vi "Additional config for txt file.vi"() -> (0 "Configuration for text file":T1)   [LabVIEW 2017]
panel:
  in  "Sweep duration (sec)":dbl=20000.0
  in  "정지":bool
  in  "Baseline Offset (pA)":dbl
  in  "Unit (A or pA)":u16(ring) items=["A", "pA"]
  in  "Sampling rate (Hz)":dbl=20000.0
  # "Please enter additional information about the data file"
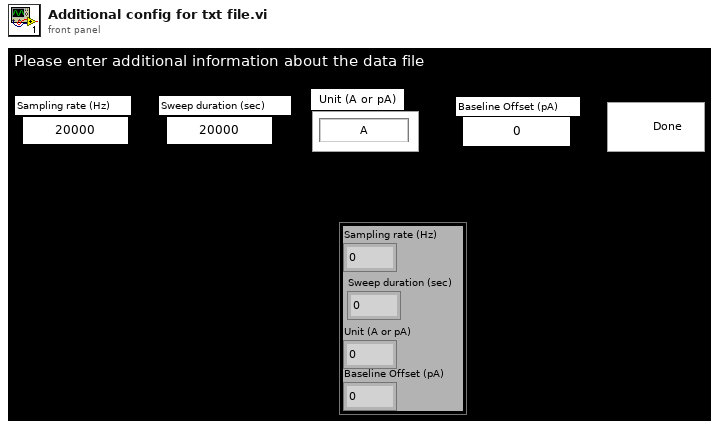
[diagram p1: front panel]
types:
  T1 = cluster{"Sampling rate (Hz)":dbl, "Sweep duration (sec)":dbl, "Unit (A or pA)":u16, "Baseline Offset (pA)":dbl}
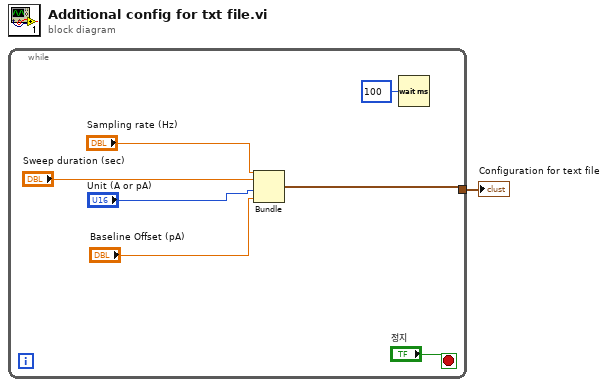
[diagram p0: block diagram]
diagram:
  n1 = while {
    tunnel: [w6] -> w1
    stop <- "정지" stop-if-true
    n2 = Bundle("Sampling rate (Hz)"="Sampling rate (Hz)", "Sweep duration (sec)"="Sweep duration (sec)", "Unit (A or pA)"="Unit (A or pA)", "Baseline Offset (pA)"="Baseline Offset (pA)") -> (w6:T1)  [unwired: 1 in]
    n3 = Wait (ms)(milliseconds to wait=u32 100 ("대기 시간 (ms)")) -> ()  [unwired: 1 out]
  }
  "Configuration for text file" <- w1
